vi "SetClassCtrl.vi"(8 "error in (no error)":errorcluster caption="entrée d'erreur (pas d'erreur)", 10 "ClassCtrlRef":refnum<vi>, 11 "EGG5210 en entrée":refnum<class "EGG5210.lvclass"> caption="DNL_LabVIEW Object in") -> (0 "error out":errorcluster caption="sortie d'erreur", 3 "EGG5210 en sortie":refnum<class "EGG5210.lvclass"> caption="DNL_LabVIEW Object out")   [LabVIEW 2012, in "EGG5210.lvclass"]
uses:
  EGG5210.lvclass
  BaseDevice/BaseDevice.lvclass
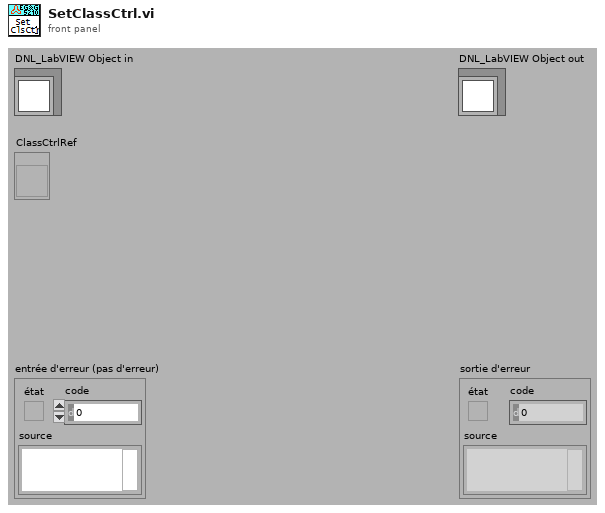
[diagram p1: front panel]
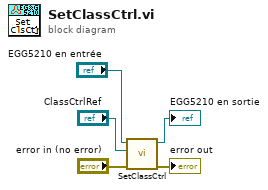
[diagram p0: block diagram]
diagram:
  n1 = call-parent "SetClassCtrl.vi"("error in (no error)"="error in (no error)", "ClassCtrlRef"="ClassCtrlRef", "BaseDevice en entrée"="EGG5210 en entrée") -> ("error out"=→"error out":errorcluster, "BaseDevice en sortie"=→"EGG5210 en sortie":refnum<class "EGG5210.lvclass">)  [unwired: 7 in]
